vi "chart axis get.vi"(8 "error in (no error)":errorcluster, 10 "axis_type":T1 items=["LXW_CHART_AXIS_TYPE_X", "LXW_CHART_AXIS_TYPE_Y", "LXW_CHART_AXIS_TYPE_X2", "LXW_CHART_AXIS_TYPE_Y2"], 11 "chart":u32) -> (0 "error out":errorcluster, 3 "function return":u32)   [LabVIEW 8.6]
doc: "lxw_chart_axis chart_axis_get(lxw_chart chart, uint8_t axis_type);"
uses:
  pending_lvxlsxwriter/xlsxwriter.dll
  Controls/lxw_chart_axis_type.ctl
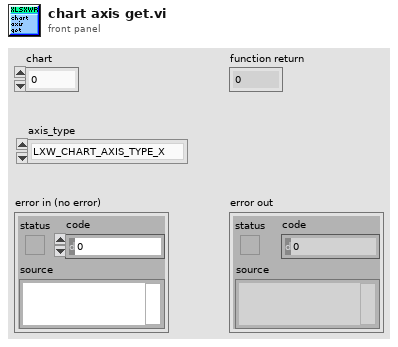
[diagram p1: front panel]
types:
  T1 = typedef "lxw_chart_axis_type.ctl" = u8
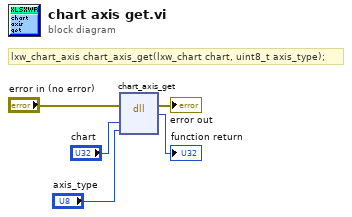
[diagram p0: block diagram]
diagram:
  # "lxw_chart_axis chart_axis_get(lxw_chart chart, uint8_t axis_type);"
  n1 = dll-call lib="C:/Users/WDAGUtilityAccount/Desktop/pending_lvxlsxwriter/xlsxwriter.*" fn="chart_axis_get"(error in="error in (no error)", "chart"="chart", "axis_type"="axis_type") -> (error out=→"error out":errorcluster, →"function return":u32)  [unwired: 4 in, 1 out]
